vi "Periodic Tasks.vi"(8 "error in":errorcluster) -> ()   [LabVIEW 2013]
doc: "This VI runs in parallel to other tasks. It can contain as many user-defined periodic loops as you need. These can carry out PID or other sorts of timed response."
uses:
  <vilib>/Rock Robotics/SystemInterfaces/Utilities/FPGA_UtilitiesLED Source.ctl
  <vilib>/Rock Robotics/SystemInterfaces/Utilities/FPGA_UtilitiesLED State.ctl
  <vilib>/Rock Robotics/WPI/DriverStation/DriverStationLCD/WPI_DriverStationLCDLCDLine.ctl
  Robot Global Data.vi
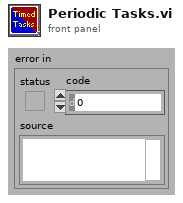
[diagram p1: front panel]
types:
  T1 = typedef "WPI_DigitalInputDevRef.ctl" = cluster{"DevStatus":errorcluster, "DIO Channel":T2, "Digital Module":T3}
  T2 = typedef "FPGA_DIOChannel.ctl" = enum8{"DIO 1", "DIO 2", "DIO 3", "DIO 4", "DIO 5", "DIO 6", "DIO 7", "DIO 8", "DIO 9", "DIO 10", "DIO 11", "DIO 12", "DIO 13", "DIO 14", "Invalid"}
  T3 = typedef "FPGA_TypedefDigitalModule.ctl" = enum16{"Digital Module 1", "Digital Module 2"}
  T4 = typedef "WPI_AnalogChannelDevRef.ctl" = cluster{"DevStatus":errorcluster, "Analog Module":T5, "Analog Channel":T6}
  T5 = typedef "FPGA_TypedefAnalogModule.ctl" = enum16{"Analog Module 1", "Analog Module 2"}
  T6 = typedef "FPGA_AIChannel.ctl" = enum8{"AI 1", "AI 2", "AI 3", "AI 4", "AI 5", "AI 6", "AI 7", "AI 8", "Invalid"}
  T7 = typedef "WPI_EncoderDevRef.ctl" = cluster{"DevStatus":errorcluster, "EncoderIndex":T8, "CounterIndex":T9, "DistancePerCount":dbl, "Decoding Type":T10}
  T8 = typedef "FPGA_EncoderIdx.ctl" = enum8{"Enc 0", "Enc 1", "Enc 2", "Enc 3", "Invalid"}
  T9 = typedef "FPGA_CounterCtrSystemIndex.ctl" = enum8{"Ctr 0", "Ctr 1", "Ctr 2", "Ctr 3", "Ctr 4", "Ctr 5", "Ctr 6", "Ctr 7", "Invalid"}
  T10 = typedef "WPI_EncoderType.ctl" = enum16{"1x", "2x", "4x"}
  T11 = cluster{"Winch Desired Location":dbl, "Winch Desired Location 2":dbl, "Winch Desired Location 3":dbl}
  T12 = typedef "FPGA_UtilitiesLED State.ctl" = enum16{"Off", "On", "Toggle"}
  T13 = typedef "FPGA_UtilitiesLED Source.ctl" = enum16{"User LED", "FPGA LED"}
  T14 = typedef "WPI_DriverStationLCDLCDLine.ctl" = enum16{"Main - Line 1", "User - Line 2", "User - Line 3", "User - Line 4", "User - Line 5", "User - Line 6"}
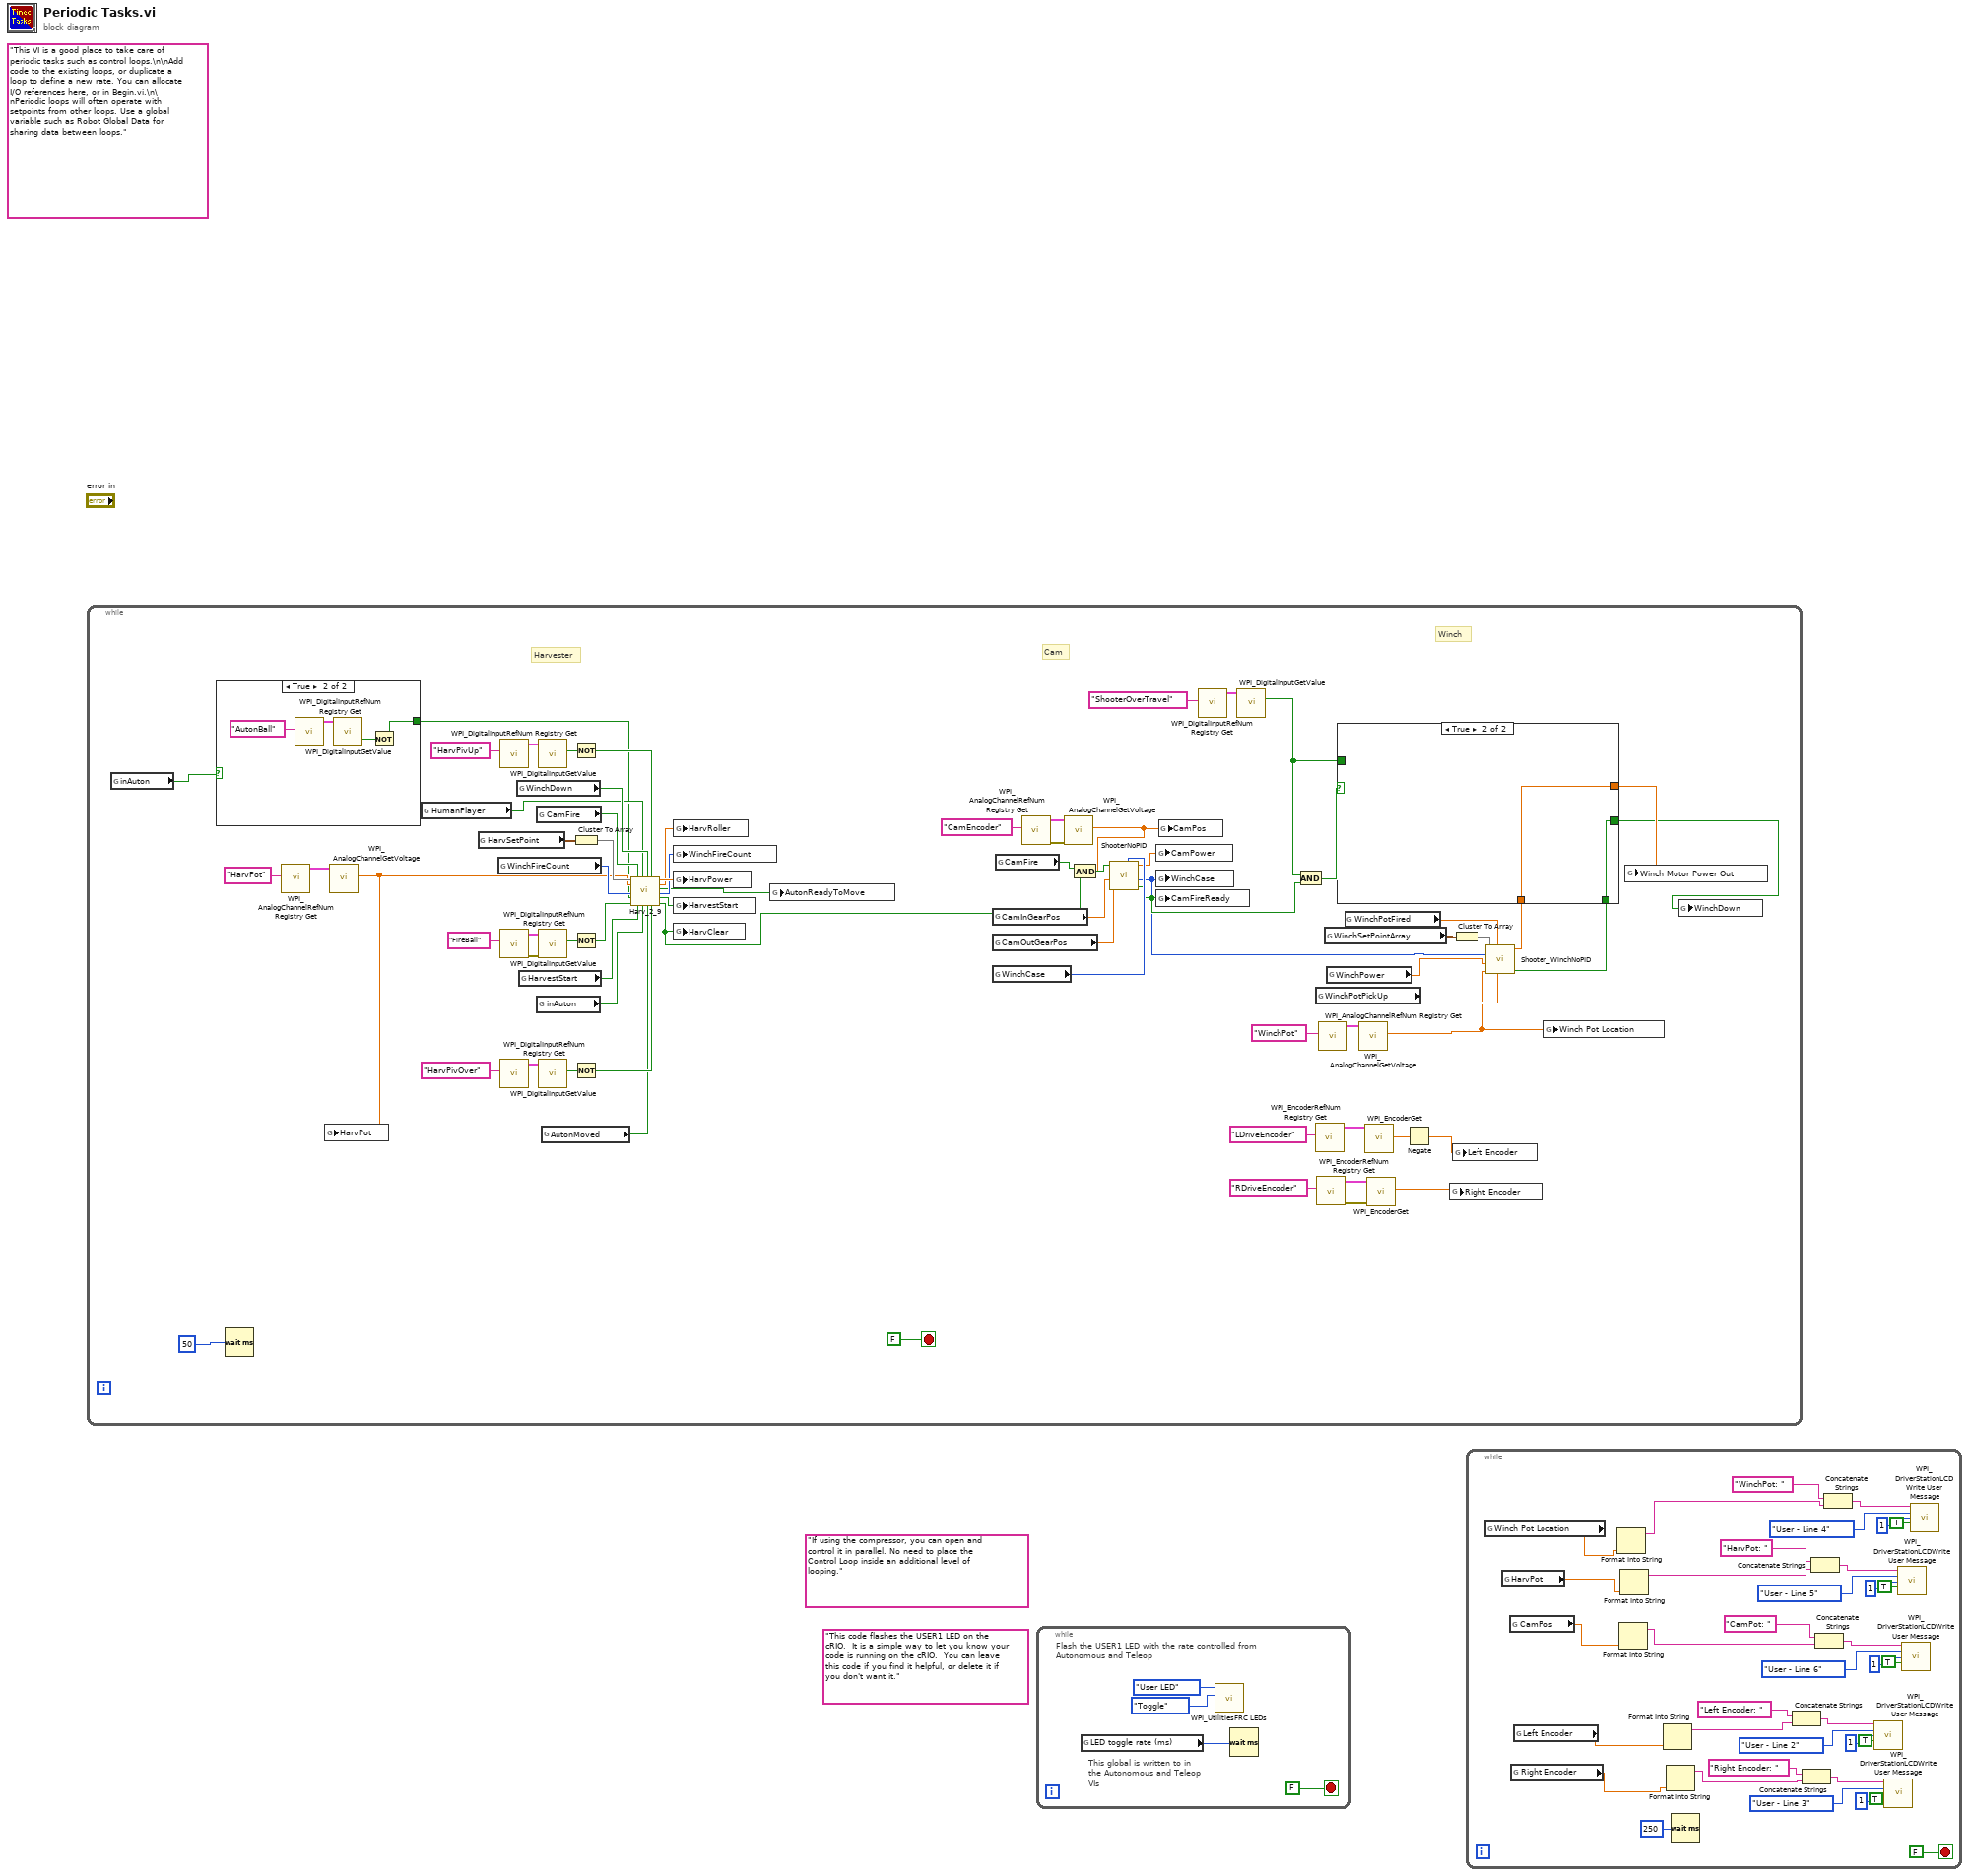
[diagram p0: block diagram]
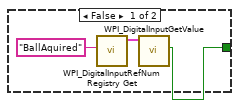
[diagram p2: hidden frame]
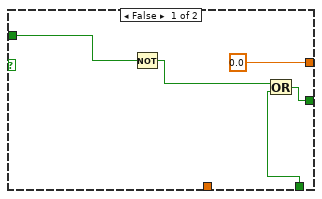
[diagram p3: hidden frame]
diagram:
  (unwired) "If using the compressor, you can open and control it in parallel. No need to place the Control Loop inside an additional level of looping."
  (unwired) "This code flashes the USER1 LED on the cRIO.  It is a simple way to let you know your code is running on the cRIO.  You can leave this code if you find it helpful, or delete it if you don't want it."
  (unwired) "This VI is a good place to take care of periodic tasks such as control loops.\n\nAdd code to the existing loops, or duplicate a loop to define a new rate. You can allocate I/O references here, or in Begin.vi.\n\nPeriodic loops will often operate with setpoints from other loops. Use a global variable such as Robot Global Data for sharing data between loops."
  n1 = while {
    stop <- FALSE stop-if-true
    # "Winch"
    # "Cam"
    # "Harvester"
    n2 = global read "Robot Global Data.vi" "inAuton"() -> (w3:bool)
    n3 = case shown="True" w3 {
      tunnel: [w72 w76] -> w2
      frame False {
        n4 = call <vilib>:"WPI_DigitalInputRefNum Registry Get.vi"("refnum name"="BallAquired") -> ("DigitalInputDevRef"=w74:T1)  [unwired: 9 in, 1 out]
        n5 = call <vilib>:"WPI_DigitalInputGetValue.vi"("DigitalInputDevRef"=w74) -> ("Value"=w72:bool)  [unwired: 8 in, 2 out]
      }
      frame True {
        n6 = call <vilib>:"WPI_DigitalInputRefNum Registry Get.vi"("refnum name"="AutonBall") -> ("DigitalInputDevRef"=w78:T1)  [unwired: 9 in, 1 out]
        n7 = call <vilib>:"WPI_DigitalInputGetValue.vi"("DigitalInputDevRef"=w78) -> ("Value"=w75:bool)  [unwired: 8 in, 2 out]
        n8 = Not(x=w75) -> (.not. x?=w76:bool)
      }
    }
    n9 = Wait (ms)(milliseconds to wait=u32 50) -> ()  [unwired: 1 out]
    n10 = call <vilib>:"WPI_AnalogChannelRefNum Registry Get.vi"("refnum name"="HarvPot") -> ("AIDeviceRef"=w70:T4)  [unwired: 9 in, 1 out]
    n11 = call <vilib>:"WPI_AnalogChannelGetVoltage.vi"("AIDeviceRef"=w70) -> ("Voltage"=w15:dbl)  [unwired: 8 in, 2 out]
    n12 = global write "Robot Global Data.vi" "HarvPot"(w15) -> ()
    n13 = global read "Robot Global Data.vi" "HumanPlayer"() -> (w6:bool)
    n14 = global read "Robot Global Data.vi" "HarvSetPoint"() -> (w41:cluster{"Out":dbl, "In":dbl, "Clear":dbl})
    n15 = global read "Robot Global Data.vi" "WinchFireCount"() -> (w18:i32)
    n16 = call <vilib>:"WPI_DigitalInputRefNum Registry Get.vi"("refnum name"="HarvPivUp") -> ("DigitalInputDevRef"=w54:T1)  [unwired: 9 in, 1 out]
    n17 = call <vilib>:"WPI_DigitalInputRefNum Registry Get.vi"("refnum name"="FireBall") -> ("error out"=w46:errorcluster, "DigitalInputDevRef"=w47:T1)  [unwired: 9 in]
    n18 = call <vilib>:"WPI_DigitalInputRefNum Registry Get.vi"("refnum name"="HarvPivOver") -> ("DigitalInputDevRef"=w62:T1)  [unwired: 9 in, 1 out]
    n19 = global read "Robot Global Data.vi" "WinchDown"() -> (w34:bool)
    n20 = global read "Robot Global Data.vi" "HarvestStart"() -> (w44:bool)
    n21 = global read "Robot Global Data.vi" "CamFire"() -> (w45:bool)
    n22 = global read "Robot Global Data.vi" "inAuton"() -> (w20:bool)
    n23 = call <vilib>:"WPI_DigitalInputGetValue.vi"("DigitalInputDevRef"=w54) -> ("Value"=w37:bool)  [unwired: 8 in, 2 out]
    n24 = call <vilib>:"WPI_DigitalInputGetValue.vi"("error in (no error)"=w46, "DigitalInputDevRef"=w47) -> ("Value"=w43:bool)  [unwired: 7 in, 2 out]
    n25 = call <vilib>:"WPI_DigitalInputGetValue.vi"("DigitalInputDevRef"=w62) -> ("Value"=w39:bool)  [unwired: 8 in, 2 out]
    n26 = global read "Robot Global Data.vi" "AutonMoved"() -> (w5:bool)
    n27 = Not(x=w37) -> (.not. x?=w36:bool)
    n28 = Cluster To Array(cluster=w41) -> (array=w40:dbl[])
    n29 = Not(x=w43) -> (.not. x?=w42:bool)
    n30 = Not(x=w39) -> (.not. x?=w38:bool)
    n31 = call "Harv_2_9.vi"("HarvSetpoints"=w40, "HarvPot"=w15, "Count"=w18, "BallAcquired"=w2, "FireBallSen"=w42, "Fire"=w45, "Harvest"=w44, "HPButton"=w6, "inAuton?"=w20, "WinchDown"=w34, "AutonMoved"=w5, "HarvPivUP"=w36, "HarvPivPickupLim"=w38) -> ("HarvPower"=w50:dbl, "HarvRoller"=w49:dbl, "AutonReadyToMove"=w4:bool, "CountOut"=w17:i32, "HarvStart"=w35:bool, "HarvCleared"=w10:bool)  [unwired: 1 in]
    n32 = global write "Robot Global Data.vi" "HarvRoller"(w49) -> ()
    n33 = global write "Robot Global Data.vi" "WinchFireCount"(w17) -> ()
    n34 = global write "Robot Global Data.vi" "HarvPower"(w50) -> ()
    n35 = global write "Robot Global Data.vi" "HarvestStart"(w35) -> ()
    n36 = global write "Robot Global Data.vi" "HarvClear"(w10) -> ()
    n37 = global write "Robot Global Data.vi" "AutonReadyToMove"(w4) -> ()
    n38 = global read "Robot Global Data.vi" "CamInGearPos"() -> (w24:dbl)
    n39 = global read "Robot Global Data.vi" "CamOutGearPos"() -> (w23:dbl)
    n40 = global read "Robot Global Data.vi" "WinchCase"() -> (w25:i32)
    n41 = global read "Robot Global Data.vi" "CamFire"() -> (w56:bool)
    n42 = call <vilib>:"WPI_AnalogChannelRefNum Registry Get.vi"("refnum name"="CamEncoder") -> ("error out"=w58:errorcluster, "AIDeviceRef"=w57:T4)  [unwired: 9 in]
    n43 = call <vilib>:"WPI_AnalogChannelGetVoltage.vi"("error in (no error)"=w58, "AIDeviceRef"=w57) -> ("Voltage"=w14:dbl)  [unwired: 7 in, 2 out]
    n44 = And(x=w56, y=w10) -> (x .and. y?=w26:bool)
    n45 = call "ShooterNoPID.vi"("WinchCaseIn"=w25, "InGearPosLow"=w23, "InGearPosHigh"=w24, "Pot"=w14, "Fire"=w26) -> ("There?"=w21:bool, "WinchCase"=w1:i32, "Power"=w22:dbl)  [unwired: 4 in]
    n46 = global write "Robot Global Data.vi" "CamPower"(w22) -> ()
    n47 = global write "Robot Global Data.vi" "WinchCase"(w1) -> ()
    n48 = global write "Robot Global Data.vi" "CamFireReady"(w21) -> ()
    n49 = global write "Robot Global Data.vi" "CamPos"(w14) -> ()
    n50 = call <vilib>:"WPI_DigitalInputRefNum Registry Get.vi"("refnum name"="ShooterOverTravel") -> ("DigitalInputDevRef"=w53:T1)  [unwired: 9 in, 1 out]
    n51 = call <vilib>:"WPI_DigitalInputGetValue.vi"("DigitalInputDevRef"=w53) -> ("Value"=w33:bool)  [unwired: 8 in, 2 out]
    n52 = And(x=w33, y=w21) -> (x .and. y?=w51:bool)
    n53 = global read "Robot Global Data.vi" "WinchPotPickUp"() -> (w19:dbl)
    n54 = call <vilib>:"WPI_EncoderRefNum Registry Get.vi"("refnum name"="LDriveEncoder") -> ("EncoderDevRef"=w64:T7)  [unwired: 9 in, 1 out]
    n55 = call <vilib>:"WPI_EncoderRefNum Registry Get.vi"("refnum name"="RDriveEncoder") -> ("error out"=w13:errorcluster, "EncoderDevRef"=w12:T7)  [unwired: 9 in]
    n56 = call <vilib>:"WPI_AnalogChannelRefNum Registry Get.vi"("refnum name"="WinchPot") -> ("AIDeviceRef"=w66:T4)  [unwired: 9 in, 1 out]
    n57 = global read "Robot Global Data.vi" "WinchSetPointArray"() -> (w30:T11)
    n58 = global read "Robot Global Data.vi" "WinchPower"() -> (w32:dbl)
    n59 = global read "Robot Global Data.vi" "WinchPotFired"() -> (w7:dbl)
    n60 = call <vilib>:"WPI_AnalogChannelGetVoltage.vi"("AIDeviceRef"=w66) -> ("Voltage"=w16:dbl)  [unwired: 8 in, 2 out]
    n61 = call <vilib>:"WPI_EncoderGet.vi"("EncoderDevRef"=w64) -> ("Distance"=w9:dbl)  [unwired: 5 in, 5 out]
    n62 = call <vilib>:"WPI_EncoderGet.vi"("error in (no error)"=w13, "EncoderDevRef"=w12) -> ("Distance"=w11:dbl)  [unwired: 4 in, 5 out]
    n63 = Negate(x=w9) -> (-x=w8:dbl)
    n64 = global write "Robot Global Data.vi" "Right Encoder"(w11) -> ()
    n65 = Cluster To Array(cluster=w30) -> (array=w31:dbl[])
    n66 = global write "Robot Global Data.vi" "Left Encoder"(w8) -> ()
    n67 = call "Shooter_WinchNoPID.vi"("PickStartPos"=w19, "WinchFiredPos"=w7, "Winch Pot Location"=w16, "WinchPower"=w32, "selectedCase"=w1, "SetPointArray"=w31) -> ("isThere?"=w28:bool, "Winch Motor Power Out"=w27:dbl)  [unwired: 4 in]
    n68 = case shown="True" w51 {
      tunnel: [0.0 ("Winch Motor Power Out") w84] -> w60
      tunnel: [w82 w85] -> w29
      tunnel: w33 -> [w81 _]
      tunnel: w28 -> [w79 w85]
      tunnel: w27 -> [_ w84]
      frame False {
        n69 = Not(x=w81) -> (.not. x?=w80:bool)
        n70 = Or(x=w80, y=w79) -> (x .or. y?=w82:bool)
      }
      frame True {
      }
    }
    n71 = global write "Robot Global Data.vi" "Winch Pot Location"(w16) -> ()
    n72 = global write "Robot Global Data.vi" "Winch Motor Power Out"(w60) -> ()
    n73 = global write "Robot Global Data.vi" "WinchDown"(w29) -> ()
  }
  n74 = while {
    stop <- FALSE stop-if-true
    # "This global is written to in the Autonomous and Teleop VIs"
    # "Flash the USER1 LED with the rate controlled from Autonomous and Teleop"
    n75 = global read "Robot Global Data.vi" "LED toggle rate (ms)"() -> (w86:u32)
    n76 = call <vilib>:"WPI_UtilitiesFRC LEDs.vi"("State"=FPGA_UtilitiesLED_State."Toggle", "LED Type"=FPGA_UtilitiesLED_Source."User LED") -> ()  [unwired: 1 in, 9 out]
    n77 = Wait (ms)(milliseconds to wait=w86) -> ()  [unwired: 1 out]
  }
  n78 = while {
    stop <- FALSE stop-if-true
    n79 = global read "Robot Global Data.vi" "Winch Pot Location"() -> (w95:dbl)
    n80 = global read "Robot Global Data.vi" "HarvPot"() -> (w94:dbl)
    n81 = global read "Robot Global Data.vi" "CamPos"() -> (w96:dbl)
    n82 = global read "Robot Global Data.vi" "Right Encoder"() -> (w92:dbl)
    n83 = global read "Robot Global Data.vi" "Left Encoder"() -> (w93:dbl)
    n84 = Format Into String(w95) -> (resulting string=w112:string)  [unwired: 3 in, 1 out]
    n85 = Format Into String(w96) -> (resulting string=w97:string)  [unwired: 3 in, 1 out]
    n86 = Format Into String(w94) -> (resulting string=w106:string)  [unwired: 3 in, 1 out]
    n87 = Format Into String(w93) -> (resulting string=w104:string)  [unwired: 3 in, 1 out]
    n88 = Format Into String(w92) -> (resulting string=w103:string)  [unwired: 3 in, 1 out]
    n89 = Wait (ms)(milliseconds to wait=u32 250) -> ()  [unwired: 1 out]
    n90 = Concatenate Strings("Left Encoder: ", w104) -> (w122:string)
    n91 = Concatenate Strings("Right Encoder: ", w103) -> (w121:string)
    n92 = Concatenate Strings("HarvPot: ", w106) -> (w107:string)
    n93 = Concatenate Strings("CamPot: ", w97) -> (w102:string)
    n94 = Concatenate Strings("WinchPot: ", w112) -> (w117:string)
    n95 = call <vilib>:"WPI_DriverStationLCDWrite User Message.vi"("line text"=w122, "line"=WPI_DriverStationLCDLCDLine."User - Line 2", "starting column"=i8 1, "clear line before write (T)"=TRUE) -> ()  [unwired: 1 in, 11 out]
    n96 = call <vilib>:"WPI_DriverStationLCDWrite User Message.vi"("line text"=w121, "line"=WPI_DriverStationLCDLCDLine."User - Line 3", "starting column"=i8 1, "clear line before write (T)"=TRUE) -> ()  [unwired: 1 in, 11 out]
    n97 = call <vilib>:"WPI_DriverStationLCDWrite User Message.vi"("line text"=w107, "line"=WPI_DriverStationLCDLCDLine."User - Line 5", "starting column"=i8 1, "clear line before write (T)"=TRUE) -> ()  [unwired: 1 in, 11 out]
    n98 = call <vilib>:"WPI_DriverStationLCDWrite User Message.vi"("line text"=w102, "line"=WPI_DriverStationLCDLCDLine."User - Line 6", "starting column"=i8 1, "clear line before write (T)"=TRUE) -> ()  [unwired: 1 in, 11 out]
    n99 = call <vilib>:"WPI_DriverStationLCDWrite User Message.vi"("line text"=w117, "line"=WPI_DriverStationLCDLCDLine."User - Line 4", "starting column"=i8 1, "clear line before write (T)"=TRUE) -> ()  [unwired: 1 in, 11 out]
  }
